vi "Multirecord Acquisition (FPGA)_20220927.vi"() -> ()   [LabVIEW 2021]
doc: "Use this VI as a template for the reconfigurable oscilloscope acquisition design. The block diagram is divided into three main loops.\n\nRegister Bus: This loop initializes the registers that are needed to support the configuration of the device. The FIFO bus, on the left, allows all the other design libraries to communicate with one another. This loop is very important to support the proper behavior of the instrument design library components.\n\nAcquisition: Acquires data from the I/O channels and writes the data into the record memory using the <B>Write</B> VI of the Multirecord Acquisition instrument design library. This VI also evaluates the various acquisition triggers and decides whether to acquire each data value in record memory. The host level VI (Fetch Record.vi) can read acquired records from the DRAM. The data is stored in 2 DRAM banks, each with 768 MB of storage.\n\nFetch: The recorded data is retrieved when the <B>Fetch Single Record</B> VI is run from the host VI. The <B>Write to Fetch DMA FIFO</B> VI writes data to the acq.fetch fifo 0 to transmit record data form the FPGA to the record fetch VIs on the host. This DMA FIFO must have a predefined name based on the instance parameter. By default, it is 0 (since the associated terminal on the <B>Create Resources DRAM Write Read</B> VI is unwired), so the connected FIFO is named acq.fetch fifo 0."
uses:
  Trigger/SubVIs/Types/Trigger Type.ctl
  <instrlib>/_niInstr/Data Trigger/v1/Shared/Public/Level Configuration FXP(+-,18,1).ctl
  <instrlib>/_niInstr/Data Trigger/v1/Shared/Public/Level Configuration Trigger When.ctl
  <instrlib>/_niInstr/Data Trigger/v1/Shared/Public/Edge Configuration FXP(+-,18,1).ctl
  <instrlib>/_niInstr/Data Trigger/v1/Shared/Public/Edge Configuration Trigger Slope.ctl
  FPGA Interface Typedefinitions/Trigger Combination Type.ctl
  <vilib>/Platform/TimedLoop/XDataNode/timing_clust.ctl
  <vilib>/Platform/TimedLoop/XDataNode/nitl_modes.ctl
  <vilib>/Platform/TimedLoop/XDataNode/wakeup.ctl
  <instrlib>/_niInstr/FIFO Register Bus/v1/FPGA/niInstr FIFO Register Bus v1 FPGA.lvclass
  C:/Program Files (x86)/National Instruments/LabVIEW 2021/instr.lib/_niInstr/Instruction Framework/v1/FPGA/Interfaces/Instruction Producer/Instruction Producer.lvclass
  <instrlib>/_niInstr/Multirecord Acquisition/Common/v1/FPGA/niInstr Multirecord Acquisition Common v1 FPGA.lvclass
  C:/Program Files (x86)/National Instruments/LabVIEW 2021/instr.lib/_niInstr/Multirecord Acquisition/Interface/v1/FPGA/niInstr Multirecord Acquisition v1 FPGA.lvclass
  <vilib>/rvi/Emulation/niFpgaSctlEmulationGetInTimedLoop.vi
  <vilib>/rvi/Emulation/niFpgaEmulationReportErrorSimple.vi
  <vilib>/rvi/Emulation/niFpgaGetClockAttributes.vi
  <vilib>/rvi/Emulation/niFpgaCriticalErrorInLSC.vi
  <instrlib>/_niInstr/Multirecord Acquisition/Common/v1/FPGA/Private/Create Fetch DMA FIFO Resources U8x32.vi
  <instrlib>/_niInstr/Multirecord Acquisition/Common/v1/FPGA/Private/Create Resources DRAM U384x2 U768 Write Read.vi
  <instrlib>/_niInstr/Multirecord Acquisition/Interface/v1/FPGA/Private/Retrieve Record U16 Wrapper.vi
  <instrlib>/_niInstr/Multirecord Acquisition/Interface/v1/FPGA/Private/Write to Fetch DMA FIFO U16 Wrapper.vi
  <vilib>/rvi/eio/common/nirviEmuTemplateMethod_errors.vi
  <instrlib>/HSAI-RIO/Config/Group A/v1/FPGA/Digital Correction/Validate 8 Channel Data.vi
  <instrlib>/HSAI-RIO/Config/Group A/v1/FPGA/Digital Correction/Digital Correction (8 Ch).vi
  <instrlib>/HSAI-RIO/Config/Group A/v1/FPGA/Digital Correction/FIR Filter (8 Ch).vi
  DSP/SubVIs/Integer decimationx8ch.vi
  Data Type Conversion/SubVIs/Remove Overflow FXP(+-,18,1)x8ch.vi
  <instrlib>/_niInstr/Channel/v1/FPGA/Private/Select/Select FXP(+-,18,1,)xNspcx8ch.vi
  Trigger/Trigger FXP(+,-,18,1).vi
  Data Type Conversion/SubVIs/Data Type Conversion FXP(+-,18,1) to I16x8ch.vi
  <instrlib>/_niInstr/Channel/v1/FPGA/Private/Select and Interleave/Select And Interleave I16xNspcx8ch.vi
  <instrlib>/_niInstr/Multirecord Acquisition/Interface/v1/FPGA/Private/Write I16 Wrapper.vi
  <vilib>/Platform/TimedLoop/XDataNode/XDataNode.xnode
  <vilib>/eio/EIONode/EIONode.xnode
  <instrlib>/_niInstr/Instruction Framework/v1/FPGA/Top Level Bus/Register Configuration/Register Configuration.lvclass
  <vilib>/Platform/TimedLoop/XDataNode/XDNodeRunTimeDep.lvlib
  <instrlib>/_niInstr/Multirecord Acquisition/Interface/v1/FPGA/niInstr Multirecord Acquisition v1 FPGA.lvclass
  <vilib>/rvi/LocalResourceManager/LocalResourceManager.xnode
  <vilib>/rvi/eio/common/nirviEmuReportErrorAndStop.vi
  <vilib>/rvi/DataTransferAndStorage/Container/Common/niFpgaContainerGetUniqueNameForEmu.vi
  <vilib>/rvi/DataTransferAndStorage/Container/Common/niFpgaContainerSetEmuInfo.vi
  <instrlib>/_niInstr/Channel/v1/FPGA/niInstr Channel v1 FPGA.lvlib
  <instrlib>/_niInstr/Basic Elements/v1/FPGA/niInstr Basic Elements v1 FPGA.lvlib
  <instrlib>/HSAI-RIO/Config/Group A/v1/FPGA/Digital Correction/Digital Correction.lvclass
  <instrlib>/HSAI-RIO/Config/Group A/v1/FPGA/Config Registers/Config Registers.lvclass
  <instrlib>/_niInstr/Data Trigger/v1/Shared/niInstr Data Trigger v1 Shared.lvlib
  C:/Program Files (x86)/National Instruments/LabVIEW 2021/instr.lib/_niInstr/Multirecord Acquisition/Common/v1/FPGA/niInstr Multirecord Acquisition Common v1 FPGA.lvclass
  <instrlib>/_niInstr/Multirecord Acquisition/Common/v1/FPGA/Private/Create Resources BRAM U384.vi
  Emulation/SubVIs/2 Element Generate Sine Cos Data FXP(+,-,14,1).vi
  <instrlib>/_niInstr/Multirecord Acquisition/Common/v1/FPGA/Private/Create Resources DRAM U384.vi
  <instrlib>/_niInstr/Multirecord Acquisition/Common/v1/FPGA/Private/Create Resources BRAM U768.vi
  FPGA Interface Typedefinitions/FPGA Interface Typedefinitions.lvlib
panel:
  in  "trigger.channel A":u8
  in  "trigger.rearm delay":u16=2
  in  "start trigger":bool=TRUE
  in  "reset":bool
  in  "trigger.combination type":T1
  in  "trigger.level B":T2
  in  "trigger.edge A":T4
  in  "trigger.level A":T2
  in  "trigger.type A":T6
  out "fifo reg bus data 0":u64
  out "fifo reg bus status 0":u32
  in  "fifo reg bus ctrl 0":u32
  out "overflow":bool
  in  "dsp.decimation factor":u16
  out "overload":bool
  in  "channel.enable mask":u16=65535 format="%.0b"
  in  "channel.number of channels":u8=8
  # "Register Bus Controls"
  # "FPGA"
  # "Acquisition Loop Controls"
  # "DSP"
  # "Trigger"
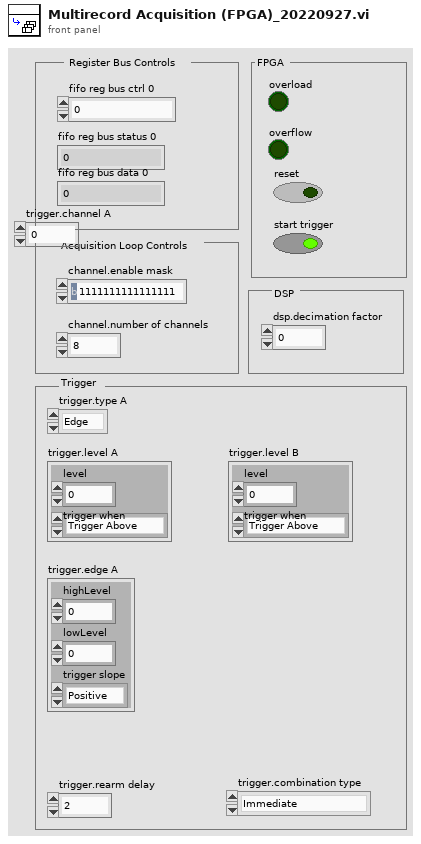
[diagram p1: front panel]
types:
  T1 = typedef "FPGA Interface Typedefinitions.lvlib/Trigger Combination Type.ctl" = enum16{"Immediate", "A", "B", "OR", "AND", "A THEN B", "B THEN A", "High Resolution"}
  T2 = typedef "niInstr Data Trigger v1 Shared.lvlib/Level Configuration FXP(+-,18,1).ctl" = cluster{"level":fxp<+/-,18,1>, "trigger when":T3}
  T3 = typedef "niInstr Data Trigger v1 Shared.lvlib/Level Configuration Trigger When.ctl" = enum8{"Trigger Above", "Trigger Below"}
  T4 = typedef "niInstr Data Trigger v1 Shared.lvlib/Edge Configuration FXP(+-,18,1).ctl" = cluster{"highLevel":fxp<+/-,18,1>, "lowLevel":fxp<+/-,18,1>, "trigger slope":T5}
  T5 = typedef "niInstr Data Trigger v1 Shared.lvlib/Edge Configuration Trigger Slope.ctl" = enum8{"Positive", "Negative"}
  T6 = typedef "Trigger Type.ctl" = enum16{"Edge", "Level", "Custom"}
  T7 = cluster{"memory 1":refnum<k21>, "memory 2":refnum<k21>}
  T8 = typedef "XDNodeRunTimeDep.lvlib/timing_clust.ctl" = cluster{"Expected End [f-1]":u64, "Actual End [f-1]":u64, "Finished Late? [f-1]":bool, "Expected End [i-1]":u64, "Actual End [i-1]":u64, "Finished Late? [i-1]":bool, "Expected Start [i]":u64, "Actual Start [i]":u64, "Expected Start [f]":u64, "Actual Start [f]":u64, "Source Name":string, "Structure Name":string, "Period":i64, "Deadline":i64, "Offset":i64, "Start":i64, "Priority":i32, "Timeout":i32, "Mode":T9, "Wakeup Reason":T10, "Error":errorcluster, "Source Type":string, "Secondary Source Type":string, "Global End Time":u64, "Global Start Time":u64, "Frame Duration":u64, "Iteration Duration":u64, "Assigned CPU":i32, "I/O Scan Engine Mode":u32}
  T9 = typedef "XDNodeRunTimeDep.lvlib/nitl_modes.ctl" = enum32{"No Change", "Process missed periods, maintain original phase", "Discard missed periods, maintain original phase", "Process missed periods, ignore original phase", "Discard missed periods, ignore original phase"}
  T10 = typedef "XDNodeRunTimeDep.lvlib/wakeup.ctl" = enum32{"Normal", "Aborted", "Asynchronous wakeup", "Timing source error", "Timed loop error", "Timeout"}
  T11 = cluster{"Channel 0":fxp<+/-,14,1>[], "Channel 1":fxp<+/-,14,1>[], "Channel 2":fxp<+/-,14,1>[], "Channel 3":fxp<+/-,14,1>[], "Channel 4":fxp<+/-,14,1>[], "Channel 5":fxp<+/-,14,1>[], "Channel 6":fxp<+/-,14,1>[], "Channel 7":fxp<+/-,14,1>[]}
  T12 = cluster{"Channel 0":fxp<+/-,18,1>[], "Channel 1":fxp<+/-,18,1>[], "Channel 2":fxp<+/-,18,1>[], "Channel 3":fxp<+/-,18,1>[], "Channel 4":fxp<+/-,18,1>[], "Channel 5":fxp<+/-,18,1>[], "Channel 6":fxp<+/-,18,1>[], "Channel 7":fxp<+/-,18,1>[]}
  T13 = cluster{"channel 0":fxp<+/-,18,1>[], "channel 1":fxp<+/-,18,1>[], "channel 2":fxp<+/-,18,1>[], "channel 3":fxp<+/-,18,1>[], "channel 4":fxp<+/-,18,1>[], "channel 5":fxp<+/-,18,1>[], "channel 6":fxp<+/-,18,1>[], "channel 7":fxp<+/-,18,1>[]}
  T14 = cluster{"channel 0":i16[], "channel 1":i16[], "channel 2":i16[], "channel 3":i16[], "channel 4":i16[], "channel 5":i16[], "channel 6":i16[], "channel 7":i16[]}
  T15 = typedef "niInstr Multirecord Acquisition v1 FPGA.lvclass/Timestamp.ctl" = cluster{"timestamp":u64, "valid":bool}
  T16 = typedef "niInstr Types v1 Shared.lvlib/Input Triggers.ctl" = cluster{"start":bool, "advance":bool, "reference":bool, "start trigger index":u16, "advance trigger index":u16, "reference trigger index":u16, "reference trigger correction cycle count":u32}
  T17 = typedef "niInstr Types v1 Shared.lvlib/Sample Format.ctl" = cluster{"bits per channel":u16, "samples per clock":u16, "channels":u8}
  T18 = typedef "niInstr Multirecord Acquisition v1 FPGA.lvclass/Events.ctl" = cluster{"ready for start":bool, "ready for advance":bool, "ready for reference":bool, "end of record":bool, "done":bool, "start trigger":bool, "advance trigger":bool, "reference trigger":bool, "start trigger index":u16, "advance trigger index":u16, "reference trigger index":u16}
  T19 = typedef "niInstr Multirecord Acquisition v1 FPGA.lvclass/Retrieve Data Info.ctl" = cluster{"read request size (bits)":u64, "valid data offset (bits)":u16, "valid data size (bits)":u16, "first sample of request":bool, "last sample of request":bool, "Token":T20}
  T20 = typedef "niInstr Types v1 Shared.lvlib/Token.ctl" = cluster{"identifier":u8, "value":u32}
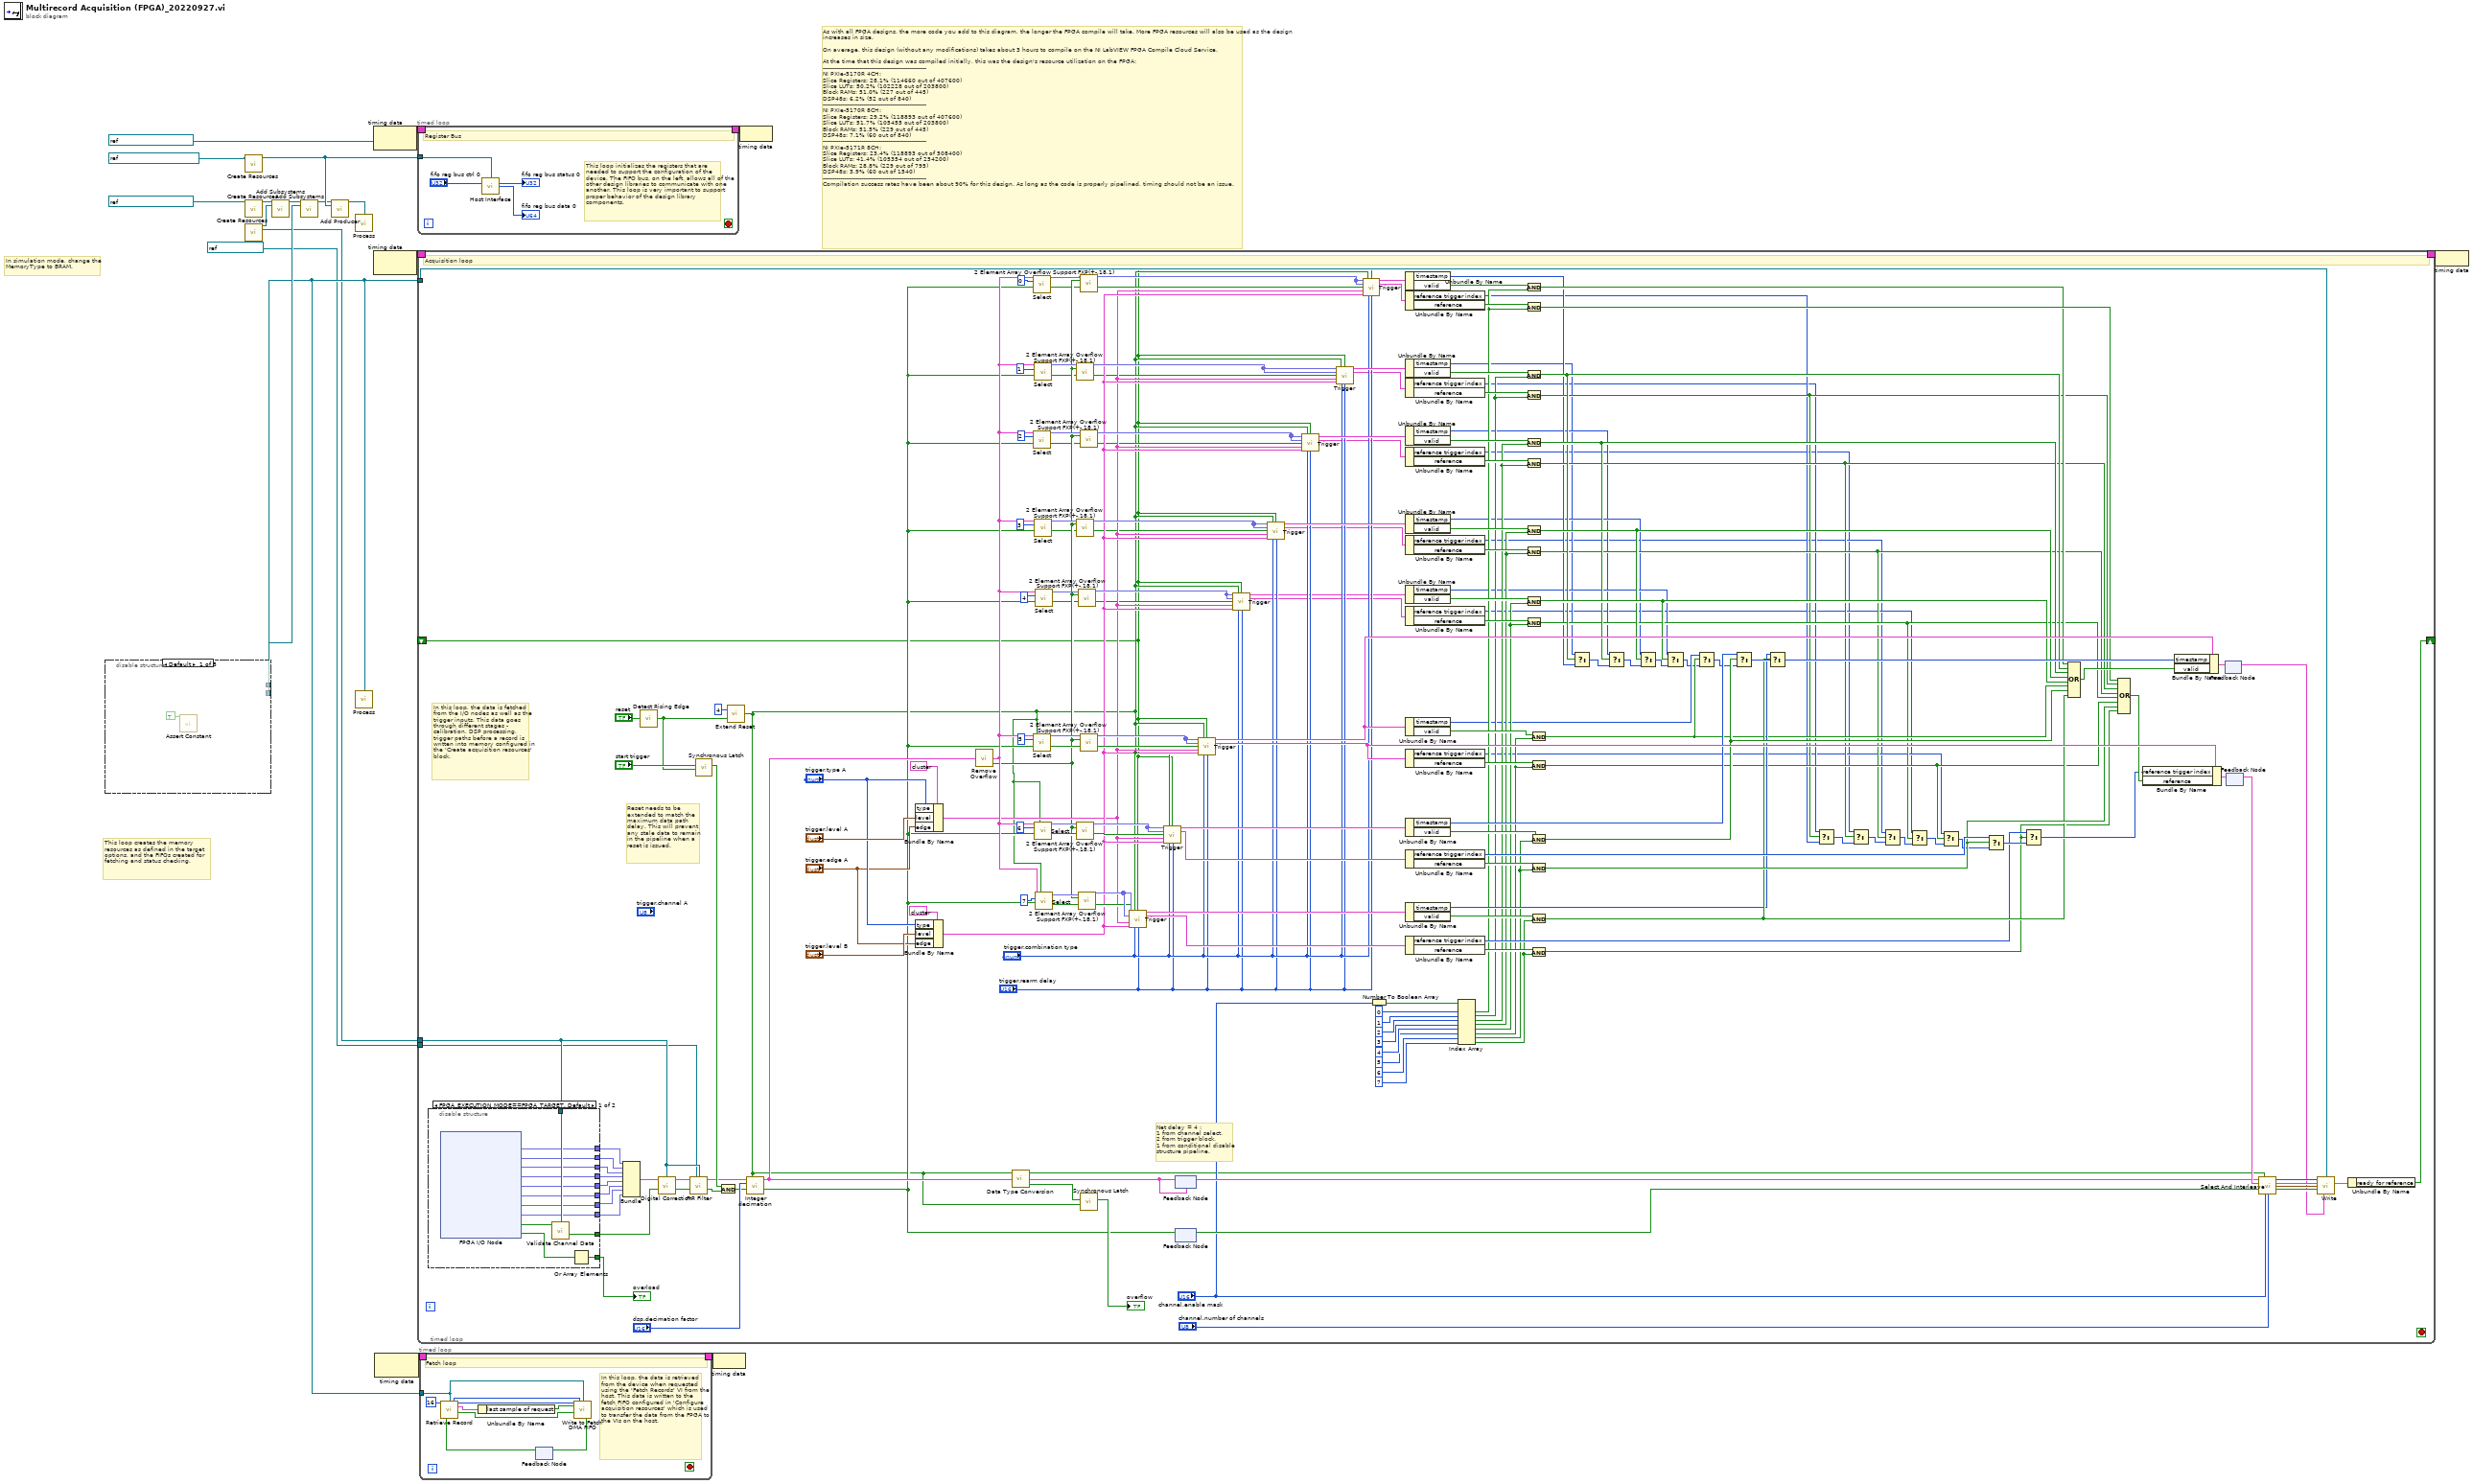
[diagram p0: block diagram]
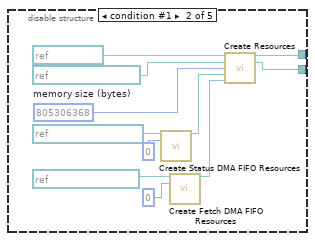
[diagram p2: hidden frame]
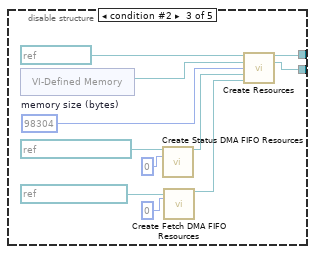
[diagram p3: hidden frame]
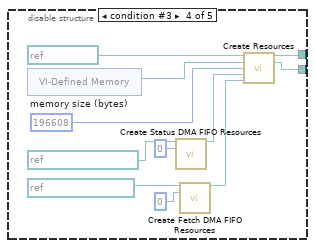
[diagram p4: hidden frame]
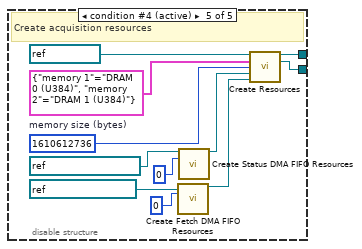
[diagram p5: hidden frame]
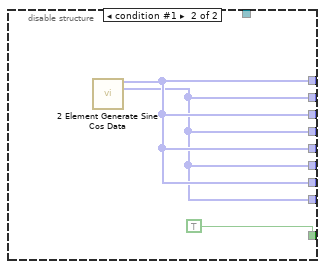
[diagram p6: hidden frame]
diagram:
  # "In simulation mode, change the MemoryType to BRAM."
  # "This loop creates the memory resources as defined in the target options, and the FIFOs created for fetching and status checking."
  # "As with all FPGA designs, the more code you add to this diagram, the longer the FPGA compile will take. More FPGA resources will also be used as the design increases in size.\n\nOn average, this design (without any modifications) takes about 3 hours to compile on the NI LabVIEW FPGA Compile Cloud Service. \n\nAt the time that this design was compiled initially, this was the design's resource utilization on the FPGA:\n------------------------------------------------------\nNI PXIe-5170R 4CH:\nSlice Registers: 28.1% (114660 out of 407600)\nSlice LUTs: 50.2% (102228 out of 203800)\nBlock RAMs: 51.0% (227 out of 445)\nDSP48s: 6.2% (52 out of 840)\n------------------------------------------------------\nNI PXIe-5170R 8CH:\nSlice Registers: 29.2% (118893 out of 407600)\nSlice LUTs: 51.7% (105455 out of 203800)\nBlock RAMs: 51.5% (229 out of 445)\nDSP48s: 7.1% (60 out of 840)\n------------------------------------------------------\nNI PXIe-5171R 8CH:\nSlice Registers: 23.4% (118893 out of 508400)\nSlice LUTs: 41.4% (105354 out of 254200)\nBlock RAMs: 28.8% (229 out of 795)\nDSP48s: 3.9% (60 out of 1540)\n------------------------------------------------------\nCompilation success rates have been about 90% for this design. As long as the code is properly pipelined, timing should not be an issue."
  n1 = disable-structure shown="Default" {
    disable-tunnel: [_ w29 w40 w51 w62] -> w4
    disable-tunnel: [_ w26 w36 w47 w59] -> w7
    frame condition #0 {
      n2 = call <instrlib>:"Assert Constant.vi"("constant terminal"=TRUE) -> ()  [unwired: 15 in]
    }
    frame condition #1 {
      w30 = u64 805306368  # memory size (bytes)
      n3 = call <instrlib>:"Create Status DMA FIFO Resources.vi"("status dma fifo in"=refnum<k21> "acq.status fifo 0" ("status dma fifo"), "fifo instance"=u8 0) -> ("status dma fifo out"=w21:refnum<class "niInstr Status FIFO v1 FPGA.lvclass">)  [unwired: 13 in]
      n4 = call-poly <instrlib>:"Create Fetch DMA FIFO Resources.vi"("fetch dma fifo in"=refnum<k21> "acq.fetch fifo 0", "fifo instance"=u8 0) -> ("fetch dma fifo out"=w27:refnum<class "niInstr Fetch FIFO v1 FPGA.lvclass">)  [unwired: 13 in]
      n5 = call-poly <instrlib>:"Create Resources.vi"("memory clock"=refnum<k21> "160MHz" ("process clock"), "memory"=refnum<k21> "DRAM 0 (U384)" ("dram"), "memory size (bytes)"=w30, "status dma fifo resources"=w21, "fetch dma fifo resources"=w27) -> ("acquisition resources"=w29:refnum<class "niInstr Multirecord Acquisition Common v1 FPGA.lvclass">, "acquisition subsystem"=w26:refnum<class "Address Space Collection.lvclass">)  [unwired: 9 in]
    }
    frame condition #2 {
      w41 = u64 98304  # memory size (bytes)
      n6 = xnode "VI-Defined Memory"() -> ("Memory Out"=w42:refnum<k21>)
      n7 = call <instrlib>:"Create Status DMA FIFO Resources.vi"("status dma fifo in"=refnum<k21> "acq.status fifo 0" ("status dma fifo"), "fifo instance"=u8 0) -> ("status dma fifo out"=w33:refnum<class "niInstr Status FIFO v1 FPGA.lvclass">)  [unwired: 13 in]
      n8 = call-poly <instrlib>:"Create Fetch DMA FIFO Resources.vi"("fetch dma fifo in"=refnum<k21> "acq.fetch fifo 0", "fifo instance"=u8 0) -> ("fetch dma fifo out"=w37:refnum<class "niInstr Fetch FIFO v1 FPGA.lvclass">)  [unwired: 13 in]
      n9 = call-poly <instrlib>:"Create Resources.vi"("memory clock"=refnum<k21> "160MHz" ("process clock"), "memory"=w42, "memory size (bytes)"=w41, "status dma fifo resources"=w33, "fetch dma fifo resources"=w37) -> ("acquisition resources"=w40:refnum<class "niInstr Multirecord Acquisition Common v1 FPGA.lvclass">, "acquisition subsystem"=w36:refnum<class "Address Space Collection.lvclass">)  [unwired: 9 in]
    }
    frame condition #3 {
      w52 = u64 196608  # memory size (bytes)
      n10 = xnode "VI-Defined Memory"() -> ("Memory Out"=w53:refnum<k21>)
      n11 = call <instrlib>:"Create Status DMA FIFO Resources.vi"("status dma fifo in"=refnum<k21> "acq.status fifo 0" ("status dma fifo"), "fifo instance"=u8 0) -> ("status dma fifo out"=w45:refnum<class "niInstr Status FIFO v1 FPGA.lvclass">)  [unwired: 13 in]
      n12 = call-poly <instrlib>:"Create Fetch DMA FIFO Resources.vi"("fetch dma fifo in"=refnum<k21> "acq.fetch fifo 0", "fifo instance"=u8 0) -> ("fetch dma fifo out"=w48:refnum<class "niInstr Fetch FIFO v1 FPGA.lvclass">)  [unwired: 13 in]
      n13 = call-poly <instrlib>:"Create Resources.vi"("memory clock"=refnum<k21> "160MHz" ("process clock"), "memory"=w53, "memory size (bytes)"=w52, "status dma fifo resources"=w45, "fetch dma fifo resources"=w48) -> ("acquisition resources"=w51:refnum<class "niInstr Multirecord Acquisition Common v1 FPGA.lvclass">, "acquisition subsystem"=w47:refnum<class "Address Space Collection.lvclass">)  [unwired: 9 in]
    }
    frame condition #4 (active) {
      w64 = u64 1610612736  # memory size (bytes)
      # "Create acquisition resources"
      n14 = call-poly <instrlib>:"Create Fetch DMA FIFO Resources.vi"("fetch dma fifo in"=refnum<k21> "acq.fetch fifo 0", "fifo instance"=u8 0) -> ("fetch dma fifo out"=w61:refnum<class "niInstr Fetch FIFO v1 FPGA.lvclass">)  [unwired: 13 in]
      n15 = call <instrlib>:"Create Status DMA FIFO Resources.vi"("status dma fifo in"=refnum<k21> "acq.status fifo 0" ("status dma fifo"), "fifo instance"=u8 0) -> ("status dma fifo out"=w56:refnum<class "niInstr Status FIFO v1 FPGA.lvclass">)  [unwired: 13 in]
      n16 = call-poly <instrlib>:"Create Resources.vi"("memory clock"=refnum<k21> "160MHz" ("process clock"), "memory"=T7 {"memory 1"="DRAM 0 (U384)", "memory 2"="DRAM 1 (U384)"}, "memory size (bytes)"=w64, "status dma fifo resources"=w56, "fetch dma fifo resources"=w61) -> ("acquisition resources"=w62:refnum<class "niInstr Multirecord Acquisition Common v1 FPGA.lvclass">, "acquisition subsystem"=w59:refnum<class "Address Space Collection.lvclass">)  [unwired: 9 in]
    }
  }
  n17 = call <instrlib>:"Create Resources.vi"("instruction fifo"=refnum<k21> "reg.host instruction fifo 0" ("FIFO")) -> ("fifo register bus"=w6:refnum<class "niInstr FIFO Register Bus v1 FPGA.lvclass">)  [unwired: 14 in]
  n18 = call <instrlib>:"Create Resources.vi"("register clock"=refnum<k21> "40 MHz Onboard Clock" ("Source Name")) -> ("register configuration"=w10:refnum<class "Register Configuration.lvclass">)  [unwired: 14 in]
  n19 = call <instrlib>:"Create Resources.vi"() -> ("config subsystems"=w8:refnum<class "Address Space Collection.lvclass">, "digital correction resources"=w1:refnum<class "Digital Correction.lvclass">)  [unwired: 14 in]
  n20 = call-dynamic "Add Subsystems.vi"("register configuration in"=w10, "subsystems"=w8) -> ("register configuration out"=w9:refnum<class "Register Configuration.lvclass">)  [unwired: 13 in]
  n21 = call-dynamic "Add Subsystems.vi"("register configuration in"=w9, "subsystems"=w7) -> ("register configuration out"=w3:refnum<class "Register Configuration.lvclass">)  [unwired: 13 in]
  n22 = call-dynamic "Add Producer.vi"("register configuration in"=w3, "instruction producer"=w6) -> ("register configuration out"=w5:refnum<class "Register Configuration.lvclass">)  [unwired: 13 in]
  n23 = call-dynamic "Process.vi"("register configuration"=w5) -> ()  [unwired: 15 in]
  n24 = call-dynamic "Process.vi"("acquisition resources"=w4) -> ()  [unwired: 15 in]
  n25 = node-c288(refnum<k21> "40 MHz Onboard Clock" ("Source Name")) -> (w19:T8)
  n26 = node-c288() -> (w17:T8)  [unwired: 1 in]
  n27 = node-c288() -> (w15:T8)  [unwired: 1 in]
  n28 = timed-loop {
    timing: w19 -> [_]
    timing-out: [_] -> w18
    tunnel: w6 -> [w68]
    stop <- _ stop-if-true
    # "This loop initializes the registers that are needed to support the configuration of the device. The FIFO bus, on the left, allows all of the other design libraries to communicate with one another. This loop is very important to support proper behavior of the design library components."
    # "Register Bus"
    n29 = call <instrlib>:"Host Interface.vi"("fifo register bus"=w68, "fifo reg bus ctrl 0"="fifo reg bus ctrl 0") -> ("fifo reg bus status 0"=→"fifo reg bus status 0":u32, "fifo reg bus data 0"=→"fifo reg bus data 0":u64)  [unwired: 12 in]
  }
  n30 = timed-loop {
    timing: w17 -> [_]
    timing-out: [_] -> w16
    tunnel: w4 -> [w256]
    tunnel: w1 -> [w235]
    shift-right: [w248] -> _
    shift-left: _ -> [w142]
    tunnel: refnum<k21> "Data Clock x2" -> [w232]
    stop <- _ stop-if-true
    # "Net delay = 4 :\n1 from channel select.\n2 from trigger block.\n1 from conditional disable structure pipeline."
    # "Reset needs to be extended to match the maximum data path delay. This will prevent any stale data to remain in the pipeline when a reset is issued."
    # "In this loop, the data is fetched from the I/O nodes as well as the trigger inputs. This data goes through different stages - calibration, DSP processing, trigger paths before a record is written into memory configured in the 'Create acquisition resources' block."
    # "Acquisition loop"
    n31 = disable-structure shown="FPGA_EXECUTION_MODE==FPGA_TARGET, Default" {
      disable-tunnel: [w268 w273] -> w231
      disable-tunnel: [w267 w272] -> w230
      disable-tunnel: [w266 w273] -> w229
      disable-tunnel: [w265 w272] -> w228
      disable-tunnel: [w264 w273] -> w227
      disable-tunnel: [w263 w272] -> w226
      disable-tunnel: [w262 w273] -> w224
      disable-tunnel: [w261 w272] -> w225
      disable-tunnel: [w258 TRUE ("ADC Data Valid")] -> w222
      disable-tunnel: w235 -> [w269 _]
      disable-tunnel: [w259 _] -> w255
      frame condition #0 (active) {
        # "I/O Nodes"
        n32 = xnode "FPGA I/O Node"() -> ("Channel 0"=w268:fxp<+/-,14,1>[], "Channel 1"=w267:fxp<+/-,14,1>[], "Channel 2"=w266:fxp<+/-,14,1>[], "Channel 3"=w265:fxp<+/-,14,1>[], "Channel 4"=w264:fxp<+/-,14,1>[], "Channel 5"=w263:fxp<+/-,14,1>[], "Channel 6"=w262:fxp<+/-,14,1>[], "Channel 7"=w261:fxp<+/-,14,1>[], "Channel Data Valid"=w270:bool[], "Channel Overload"=w260:bool[])  [unwired: 10 in, 10 out]
        n33 = call-poly <instrlib>:"Validate Channel Data.vi"("channel data valid"=w270, "digital correction resources"=w269) -> ("expected data valid"=w258:bool)  [unwired: 13 in]
        n34 = Or Array Elements(Boolean array=w260) -> (logical OR=w259:bool)
      }
      frame condition #1 {
        n35 = call-poly "2 Element Generate Sine Cos Data.vi"() -> ("sine data"=w273:fxp<+/-,14,1>[], "cosine data"=w272:fxp<+/-,14,1>[])  [unwired: 14 in]
      }
    }
    "overload" <- w255
    n36 = Bundle("Channel 0"=w231, "Channel 1"=w230, "Channel 2"=w229, "Channel 3"=w228, "Channel 4"=w227, "Channel 5"=w226, "Channel 6"=w224, "Channel 7"=w225) -> (w223:T11)  [unwired: 1 in]
    n37 = call <instrlib>:"Detect Rising Edge.vi"("signal"="reset") -> ("edge detected"=w234:bool)  [unwired: 14 in]
    n38 = call-poly <instrlib>:"Digital Correction.vi"("channel data in"=w223, "digital correction resources"=w235, "input valid"=w222) -> ("corrected channel data out"=w215:T12, "output valid"=w214:bool)  [unwired: 11 in]
    n39 = call-poly <instrlib>:"FIR Filter.vi"("data in"=w215, "data clock x2"=w232, "digital correction resources"=w235, "input valid"=w214) -> ("data out"=w212:T12, "output valid"=w213:bool)  [unwired: 9 in, 1 out]
    n40 = call <instrlib>:"Synchronous Latch.vi"("clear"=w234, "set"="start trigger") -> ("out"=w240:bool)  [unwired: 9 in]
    n41 = And(x=w240, y=w213) -> (x .and. y?=w216:bool)
    n42 = call "Extend Reset.vi"("reset in"=w234, "number of cycles"=u8 4) -> ("reset out"=w143:bool)
    n43 = call-poly "Integer decimation.vi"("data in"=w212, "reset"=w143, "decimation factor"="dsp.decimation factor", "input valid"=w216) -> ("data out"=w219:T13, "output valid"=w161:bool)  [unwired: 9 in, 1 out]
    n44 = Bundle By Name(cluster=cluster{"type":T6, "level":T2, "edge":T4} {"type"=enum."Edge", "level"={"level"=0.0, "trigger when"=enum."Trigger Above"}, "edge"={"highLevel"=0.0, "lowLevel"=0.0, "trigger slope"=enum."Positive"}} ("trigger.A"), "type"="trigger.type A", "level"="trigger.level A", "edge"="trigger.edge A") -> (w154:cluster{"type":T6, "level":T2, "edge":T4})
    n45 = Bundle By Name(cluster=cluster{"type":T6, "level":T2, "edge":T4} {"type"=enum."Edge", "level"={"level"=0.0, "trigger when"=enum."Trigger Above"}, "edge"={"highLevel"=0.0, "lowLevel"=0.0, "trigger slope"=enum."Positive"}} ("trigger.A"), "type"="trigger.type A", "level"="trigger.level B", "edge"="trigger.edge A") -> (w155:cluster{"type":T6, "level":T2, "edge":T4})
    n46 = call-poly "Remove Overflow.vi"("data in"=w219) -> ("overflow"=w153:bool, "data out"=w167:T13)  [unwired: 3 in]
    n47 = call-poly "Data Type Conversion.vi"("data in"=w219) -> ("overflow"=w221:bool, "data out"=w218:T14)  [unwired: 3 in]
    n48 = call-poly <instrlib>:"Select.vi"("data in"=w167, "channel index"=u8 0 ("trigger.channel A"), "input valid"=w161) -> ("channel out"=w166:fxp<+/-,18,1>[], "output valid"=w148:bool)  [unwired: 11 in]
    n49 = call-poly <instrlib>:"Select.vi"("data in"=w167, "channel index"=u8 2 ("trigger.channel A"), "input valid"=w161) -> ("channel out"=w164:fxp<+/-,18,1>[], "output valid"=w150:bool)  [unwired: 11 in]
    n50 = call-poly <instrlib>:"Select.vi"("data in"=w167, "reset"=w143, "channel index"=u8 5 ("trigger.channel A"), "input valid"=w161) -> ("channel out"=w242:fxp<+/-,18,1>[], "output valid"=w211:bool)  [unwired: 10 in]
    n51 = call-poly <instrlib>:"Select.vi"("data in"=w167, "channel index"=u8 1, "input valid"=w161) -> ("channel out"=w165:fxp<+/-,18,1>[], "output valid"=w149:bool)  [unwired: 11 in]
    n52 = call-poly <instrlib>:"Select.vi"("data in"=w167, "channel index"=u8 3, "input valid"=w161) -> ("channel out"=w163:fxp<+/-,18,1>[], "output valid"=w151:bool)  [unwired: 11 in]
    n53 = call-poly <instrlib>:"Select.vi"("data in"=w167, "reset"=w143, "channel index"=u8 6, "input valid"=w161) -> ("channel out"=w206:fxp<+/-,18,1>[], "output valid"=w204:bool)  [unwired: 10 in]
    n54 = call-poly <instrlib>:"Select.vi"("data in"=w167, "channel index"=u8 4, "input valid"=w161) -> ("channel out"=w162:fxp<+/-,18,1>[], "output valid"=w152:bool)  [unwired: 11 in]
    n55 = call-poly <instrlib>:"Select.vi"("data in"=w167, "reset"=w143, "channel index"=u8 7, "input valid"=w161) -> ("channel out"=w185:fxp<+/-,18,1>[], "output valid"=w183:bool)  [unwired: 10 in]
    n56 = call "2 Element Array Overflow Support FXP(+-,18,1).vi"("data in"=w165, "overflow"=w153) -> ("data out"=w159:fxp<+/-,18,1>[])  [unwired: 13 in]
    n57 = call "2 Element Array Overflow Support FXP(+-,18,1).vi"("data in"=w163, "overflow"=w153) -> ("data out"=w157:fxp<+/-,18,1>[])  [unwired: 13 in]
    n58 = call "2 Element Array Overflow Support FXP(+-,18,1).vi"("data in"=w206, "overflow"=w153) -> ("data out"=w205:fxp<+/-,18,1>[])  [unwired: 13 in]
    n59 = call "2 Element Array Overflow Support FXP(+-,18,1).vi"("data in"=w162, "overflow"=w153) -> ("data out"=w156:fxp<+/-,18,1>[])  [unwired: 13 in]
    n60 = call "2 Element Array Overflow Support FXP(+-,18,1).vi"("data in"=w185, "overflow"=w153) -> ("data out"=w184:fxp<+/-,18,1>[])  [unwired: 13 in]
    n61 = call "2 Element Array Overflow Support FXP(+-,18,1).vi"("data in"=w166, "overflow"=w153) -> ("data out"=w160:fxp<+/-,18,1>[])  [unwired: 13 in]
    n62 = call "2 Element Array Overflow Support FXP(+-,18,1).vi"("data in"=w164, "overflow"=w153) -> ("data out"=w158:fxp<+/-,18,1>[])  [unwired: 13 in]
    n63 = call "2 Element Array Overflow Support FXP(+-,18,1).vi"("data in"=w242, "overflow"=w153) -> ("data out"=w210:fxp<+/-,18,1>[])  [unwired: 13 in]
    n64 = call <instrlib>:"Synchronous Latch.vi"("clear"=w143, "set"=w221) -> ("out"=→"overflow":bool)  [unwired: 9 in]
    n65 = call-poly "Trigger.vi"("data A"=w184, "reset"=w143, "trigger.ready for reference"=w142, "data B"=w184, "input valid"=w183, "trigger.A"=w154, "trigger.B"=w155, "trigger.combination type"="trigger.combination type", "rearm delay"="trigger.rearm delay") -> ("timestamps"=w182:T15, "trigger.out"=w181:T16)  [unwired: 4 in, 1 out]
    n66 = call-poly "Trigger.vi"("data A"=w205, "reset"=w143, "trigger.ready for reference"=w142, "data B"=w205, "input valid"=w204, "trigger.A"=w154, "trigger.B"=w155, "trigger.combination type"="trigger.combination type", "rearm delay"="trigger.rearm delay") -> ("timestamps"=w199:T15, "trigger.out"=w198:T16)  [unwired: 4 in, 1 out]
    n67 = feedback #1(w218) -> (w220:T14)
    n68 = feedback-in #1(w218) -> ()
    n69 = feedback #2() -> (w217:bool)  [unwired: 1 in]
    n70 = feedback-in #2(w161) -> ()
    n71 = call-poly "Trigger.vi"("data A"=w210, "reset"=w143, "trigger.ready for reference"=w142, "data B"=w210, "input valid"=w211, "trigger.A"=w154, "trigger.B"=w155, "trigger.combination type"="trigger.combination type", "rearm delay"="trigger.rearm delay") -> ("timestamps"=w203:T15, "trigger.out"=w201:T16)  [unwired: 4 in, 1 out]
    n72 = call-poly "Trigger.vi"("data A"=w156, "reset"=w143, "trigger.ready for reference"=w142, "data B"=w156, "input valid"=w152, "trigger.A"=w154, "trigger.B"=w155, "trigger.combination type"="trigger.combination type", "rearm delay"="trigger.rearm delay") -> ("timestamps"=w135:T15, "trigger.out"=w134:T16)  [unwired: 4 in, 1 out]
    n73 = call-poly "Trigger.vi"("data A"=w157, "reset"=w143, "trigger.ready for reference"=w142, "data B"=w157, "input valid"=w151, "trigger.A"=w154, "trigger.B"=w155, "trigger.combination type"="trigger.combination type", "rearm delay"="trigger.rearm delay") -> ("timestamps"=w144:T15, "trigger.out"=w136:T16)  [unwired: 4 in, 1 out]
    n74 = call-poly "Trigger.vi"("data A"=w158, "reset"=w143, "trigger.ready for reference"=w142, "data B"=w158, "input valid"=w150, "trigger.A"=w154, "trigger.B"=w155, "trigger.combination type"="trigger.combination type", "rearm delay"="trigger.rearm delay") -> ("timestamps"=w145:T15, "trigger.out"=w137:T16)  [unwired: 4 in, 1 out]
    n75 = call-poly "Trigger.vi"("data A"=w159, "reset"=w143, "trigger.ready for reference"=w142, "data B"=w159, "input valid"=w149, "trigger.A"=w154, "trigger.B"=w155, "trigger.combination type"="trigger.combination type", "rearm delay"="trigger.rearm delay") -> ("timestamps"=w146:T15, "trigger.out"=w138:T16)  [unwired: 4 in, 1 out]
    n76 = call-poly "Trigger.vi"("data A"=w160, "reset"=w143, "trigger.ready for reference"=w142, "data B"=w160, "input valid"=w148, "trigger.A"=w154, "trigger.B"=w155, "trigger.combination type"="trigger.combination type", "rearm delay"="trigger.rearm delay") -> ("timestamps"=w147:T15, "trigger.out"=w139:T16)  [unwired: 4 in, 1 out]
    n77 = Number To Boolean Array(number="channel.enable mask") -> (Boolean array=w194:bool[])
    n78 = Unbundle By Name(w147) -> ("timestamp"=w97:u64, "valid"=w128:bool)
    n79 = Unbundle By Name(w139) -> ("reference trigger index"=w86:u16, "reference"=w127:bool)
    n80 = Unbundle By Name(w146) -> ("timestamp"=w87:u64, "valid"=w126:bool)
    n81 = Unbundle By Name(w138) -> ("reference trigger index"=w85:u16, "reference"=w125:bool)
    n82 = Unbundle By Name(w145) -> ("timestamp"=w88:u64, "valid"=w124:bool)
    n83 = Unbundle By Name(w137) -> ("reference trigger index"=w76:u16, "reference"=w123:bool)
    n84 = Unbundle By Name(w144) -> ("timestamp"=w89:u64, "valid"=w122:bool)
    n85 = Unbundle By Name(w136) -> ("reference trigger index"=w77:u16, "reference"=w121:bool)
    n86 = Unbundle By Name(w135) -> ("timestamp"=w90:u64, "valid"=w120:bool)
    n87 = Unbundle By Name(w134) -> ("reference trigger index"=w78:u16, "reference"=w119:bool)
    n88 = Unbundle By Name(w203) -> ("timestamp"=w96:u64, "valid"=w191:bool)
    n89 = Unbundle By Name(w201) -> ("reference trigger index"=w80:u16, "reference"=w189:bool)
    n90 = Unbundle By Name(w199) -> ("timestamp"=w197:u64, "valid"=w190:bool)
    n91 = Unbundle By Name(w198) -> ("reference trigger index"=w196:u16, "reference"=w188:bool)
    n92 = Unbundle By Name(w182) -> ("timestamp"=w169:u64, "valid"=w179:bool)
    n93 = Unbundle By Name(w181) -> ("reference trigger index"=w168:u16, "reference"=w180:bool)
    n94 = Index Array(array=w194, index #1=0 ("index"), index #2=1 ("index"), index #3=2 ("index"), index #4=3 ("index"), index #5=4 ("index"), index #6=5 ("index"), index #7=6 ("index"), index #8=7 ("index")) -> (element #1=w118:bool, element #2=w117:bool, element #3=w116:bool, element #4=w115:bool, element #5=w114:bool, element #6=w113:bool, element #7=w112:bool, element #8=w111:bool)
    n95 = And(x=w128, y=w118) -> (x .and. y?=w108:bool)
    n96 = And(x=w127, y=w118) -> (x .and. y?=w109:bool)
    n97 = And(x=w126, y=w117) -> (x .and. y?=w103:bool)
    n98 = And(x=w125, y=w117) -> (x .and. y?=w98:bool)
    n99 = And(x=w124, y=w116) -> (x .and. y?=w104:bool)
    n100 = And(x=w123, y=w116) -> (x .and. y?=w99:bool)
    n101 = And(x=w122, y=w115) -> (x .and. y?=w105:bool)
    n102 = And(x=w121, y=w115) -> (x .and. y?=w100:bool)
    n103 = And(x=w120, y=w114) -> (x .and. y?=w106:bool)
    n104 = And(x=w119, y=w114) -> (x .and. y?=w101:bool)
    n105 = And(x=w191, y=w113) -> (x .and. y?=w107:bool)
    n106 = And(x=w189, y=w113) -> (x .and. y?=w102:bool)
    n107 = And(x=w190, y=w112) -> (x .and. y?=w178:bool)
    n108 = And(x=w188, y=w112) -> (x .and. y?=w176:bool)
    n109 = And(x=w179, y=w111) -> (x .and. y?=w170:bool)
    n110 = And(x=w180, y=w111) -> (x .and. y?=w110:bool)
    n111 = Select(t=w87, s=w103, f=w97) -> (s? t:f=w91:u64)
    n112 = Select(t=w88, s=w104, f=w91) -> (s? t:f=w92:u64)
    n113 = Select(t=w89, s=w105, f=w92) -> (s? t:f=w93:u64)
    n114 = Select(t=w90, s=w106, f=w93) -> (s? t:f=w94:u64)
    n115 = Select(t=w96, s=w107, f=w94) -> (s? t:f=w95:u64)
    n116 = Select(t=w197, s=w178, f=w95) -> (s? t:f=w174:u64)
    n117 = Select(t=w169, s=w170, f=w174) -> (s? t:f=w173:u64)
    n118 = Select(t=w85, s=w98, f=w86) -> (s? t:f=w84:u16)
    n119 = Select(t=w76, s=w99, f=w84) -> (s? t:f=w83:u16)
    n120 = Select(t=w77, s=w100, f=w83) -> (s? t:f=w82:u16)
    n121 = Select(t=w78, s=w101, f=w82) -> (s? t:f=w81:u16)
    n122 = Select(t=w80, s=w102, f=w81) -> (s? t:f=w79:u16)
    n123 = Select(t=w196, s=w176, f=w79) -> (s? t:f=w172:u16)
    n124 = Select(t=w168, s=w110, f=w172) -> (s? t:f=w171:u16)
    n125 = Compound Arithmetic op=OR(w108, w103, w104, w105, w106, w107, w178, w170) -> (w177:bool)
    n126 = Compound Arithmetic op=OR(w109, w98, w99, w100, w101, w102, w176, w110) -> (w175:bool)
    n127 = Bundle By Name(cluster=w201, "reference trigger index"=w171, "reference"=w175) -> (w200:T16)
    n128 = Bundle By Name(cluster=w203, "timestamp"=w173, "valid"=w177) -> (w202:T15)
    n129 = feedback #3() -> (w238:T15)  [unwired: 1 in]
    n130 = feedback-in #3(w202) -> ()
    n131 = feedback #4() -> (w239:T16)  [unwired: 1 in]
    n132 = feedback-in #4(w200) -> ()
    n133 = call-poly <instrlib>:"Select And Interleave.vi"("data in"=w220, "reset"=w143, "triggers in"=w239, "input valid"=w217, "channel enable mask"="channel.enable mask", "number of channels to interleave"="channel.number of channels") -> ("interleaved data out"=w254:i16[], "triggers out"=w253:T16, "sample format out"=w252:T17, "output valid"=w251:bool)  [unwired: 5 in, 1 out]
    n134 = call-poly <instrlib>:"Write.vi"("data"=w254, "acquisition resources"=w256, "triggers"=w253, "sample format"=w252, "data valid"=w251, "timestamp"=w238) -> ("events"=w249:T18)  [unwired: 6 in, 3 out]
    n135 = Unbundle By Name(w249) -> ("ready for reference"=w248:bool)
  }
  n136 = timed-loop {
    timing: w15 -> [_]
    timing-out: [_] -> w14
    tunnel: w4 -> [w284]
    stop <- _ stop-if-true
    # "In this loop, the data is retrieved from the device when requested using the 'Fetch Records' VI from the host. This data is written to the fetch FIFO configured in 'Configure acquisition resources' which is used to transfer the data from the FPGA to the VIs on the host."
    # "Fetch loop"
    n137 = feedback #5() -> (w282:bool)  [unwired: 1 in]
    n138 = call-poly <instrlib>:"Retrieve Record.vi"("output array size"=u16 16, "acquisition resources"=w284, "ready for output"=w282) -> ("channels"=w277:u8, "data"=w280:u16[], "retrieve data info"=w279:T19, "output valid"=w281:bool)  [unwired: 9 in]
    n139 = Unbundle By Name(w279) -> ("last sample of request"=w278:bool)
    n140 = call-poly <instrlib>:"Write to Fetch DMA FIFO.vi"("data"=w280, "channels"=w277, "acquisition resources"=w284, "last sample of request"=w278, "input valid"=w281) -> ("ready for input"=w283:bool)  [unwired: 10 in]
    n141 = feedback-in #5(w283) -> ()
  }
  n142 = node-c288(w14) -> ()
  n143 = node-c288(w18) -> ()
  n144 = node-c288(w16) -> ()
